vi "Phase III PID.vi"() -> ()   [LabVIEW 2022 SP3]
uses:
  Controls/Notifier data ctl.ctl
  Globals/Phase III Globals.vi
panel:
  out "E_TC_NE":dbl format="%.2g"
  out "E_TC_ET2":dbl format="%.2g"
  out "N_EPV_202_NO":bool
  out "Boolean 92":bool
  out "Boolean 93":bool
  out "Boolean 91":bool
  out "E_PT_CC1":dbl format="%.2g"
  out "E_RTD_NE2":dbl format="%.2g"
  out "E_RTD_NE1":dbl format="%.2g"
  out "E_RTD_ET2":dbl format="%.2g"
  out "E_RTD_ET1":dbl format="%.2g"
  out "E_RTD_TC2":dbl format="%.2g"
  out "E_RTD_TC1":dbl format="%.2g"
  out "Boolean 90":bool
  out "Boolean 89":bool
  out "Boolean 88":bool
  out "F_PT_32":dbl format="%.2g"
  out "C_PT_156":dbl format="%.2g"
  in  "notifier out":refnum<notifier>
  out "F_EPV_136 _NC":bool
  out "F_EPV_41_NC":bool
  out "N_EPV_75_NO":bool
  out "N_EPV_75_NO HS":bool
  out "N_EPV_203_NO":bool
  out "F_EPV_28_NC":bool
  out "F_EPV_1352_NO":bool
  out "N_EPV_62a_NO":bool
  out "C_EPV_7_NC":bool
  out "C_EPV_ 2_NC":bool
  out "F_CMFM_27 (FR)":dbl format="%.2g"
  out "Boolean 87":bool
  out "F_CMFM_43(D)":dbl format="%.2g"
  out "C_CMFM_11 (D)":dbl format="%.2g"
  out "G_CMFM_53 (FR)":dbl format="%.2g"
  out "Boolean 38":bool
  out "C_EPV_ 141_NO HS":bool
  out "N_EPV_69_NO":bool
  out "Boolean 3":bool
  out "N_EPV_68_NO":bool
  out "N_EPV_68_NO HS":bool
  out "Boolean 6":bool
  out "F_EPV_131_NO":bool
  out "Boolean 18":bool
  out "G_EPV_51_NC":bool
  out "C_EPV_ 124_NO":bool
  out "Boolean 13":bool
  out "N_EPV_142_NO":bool
  out "Boolean 41":bool
  out "Boolean 11":bool
  out "Boolean 14":bool
  out "Boolean 29":bool
  out "Boolean 28":bool
  out "Boolean 27":bool
  out "Boolean 26":bool
  out "Boolean 25":bool
  out "Boolean 9":bool
  out "Boolean 7":bool
  out "Boolean 8":bool
  out "Boolean 5":bool
  out "Boolean 6":bool
  out "Boolean 3":bool
  out "Boolean 4":bool
  out "Boolean 24":bool
  out "Boolean 23":bool
  out "Boolean 25":bool
  out "Boolean 26":bool
  out "Boolean 21":bool
  out "N_EPV_61_NO":bool
  out "I_Voltage(V)":dbl format="%.2g"
  out "I_Current(A)":dbl format="%.2g"
  out "Boolean 724":bool
  out "F_CMFM_43(FR)":dbl format="%.2g"
  out "C_PT_45":dbl format="%.2g"
  out "G_CMFM_53(D)":dbl format="%.2g"
  out "C_PT_55":dbl format="%.2g"
  out "C_RTD_20":dbl format="%.2g"
  out "Boolean 18":bool
  out "Boolean 36":bool
  out "Boolean 47":bool
  out "Boolean 4":bool
  out "C_EPV_7_NC HS":bool
  out "Boolean 14":bool
  out "Boolean 19":bool
  out "Boolean 31":bool
  out "Boolean 30":bool
  out "Boolean 24":bool
  out "Boolean 35":bool
  out "Boolean 33":bool
  out "Boolean 34":bool
  out "Boolean 32":bool
  out "Boolean 10":bool
  out "Boolean 11":bool
  out "Boolean 12":bool
  out "Boolean 6":bool
  out "Boolean 45":bool
  out "Boolean 44":bool
  out "Boolean 46":bool
  out "Boolean 42":bool
  out "Boolean 40":bool
  out "Boolean 39":bool
  out "N_EPV_142_NO HS":bool
  out "Boolean 37":bool
  out "Boolean 43":bool
  out "Boolean38":bool
  out "Boolean 7":bool
  out "Boolean 1":bool
  out "Boolean 2":bool
  out "N_EPV_69_NO HS":bool
  out "Boolean 4":bool
  out "Boolean 9":bool
  out "Boolean 5":bool
  out "Boolean 8":bool
  out "Boolean 10":bool
  out "Boolean 11":bool
  out "Boolean 12":bool
  out "Boolean 18":bool
  out "Boolean 13":bool
  out "Boolean 17":bool
  out "Boolean 16":bool
  out "Boolean 19":bool
  out "Boolean 9":bool
  out "Boolean 8":bool
  out "N_EPV_206_NO":bool
  out "Boolean 16":bool
  out "Boolean 15":bool
  out "N_EPV_206_NO HS":bool
  out "Boolean 23":bool
  out "Boolean 22":bool
  out "Boolean 21":bool
  out "Boolean 17":bool
  out "N_EPV_203_NO HS":bool
  out "Boolean 13":bool
  out "Boolean 12":bool
  out "Boolean 27":bool
  out "Boolean 26":bool
  out "Boolean":bool
  out "F_PT_49":dbl format="%.2g"
  out "Boolean 23":bool
  out "Boolean 24":bool
  out "F_EPV_41_NC HS":bool
  out "Boolean 22":bool
  out "Boolean 21":bool
  out "Boolean 20":bool
  out "Boolean 15":bool
  out "Boolean 10":bool
  out "Boolean 1":bool
  out "Boolean 2":bool
  out "I_MPT":dbl format="%.2g"
  out "C_PT_13d":dbl format="%.2g"
  out "C_RTD_13b":dbl format="%.2g"
  out "C_PT_13b":dbl format="%.2g"
  out "Boolean 4":bool
  out "Boolean 18":bool
  out "F_RTD_31a":dbl format="%.2g"
  out "F_PT_31a":dbl format="%.2g"
  out "Boolean 3":bool
  out "Boolean 5":bool
  out "Boolean 2":bool
  out "Boolean 1":bool
  out "E_TC_CC":dbl format="%.2g"
  out "F_RTD_Regen1":dbl format="%.2g"
  out "F_RTD_Regen2":dbl format="%.2g"
  out "E_TC_ET":dbl format="%.2g"
  out "Boolean 9":bool caption="Boolean 6"
  out "Boolean 8":bool
  out "F_PT_29 a":dbl format="%.2g"
  out "F_RTD_29":dbl format="%.2g"
  out "Boolean 7":bool
  out "F_EPV_28_NC HS":bool
  out "F_PT_D":dbl format="%.2g"
  out "Boolean 5":bool
  out "F_PT_SC":dbl format="%.2g"
  out "F_RTD_SC":dbl format="%.2g"
  out "F_PT_S":dbl format="%.2g"
  out "Boolean 4":bool
  out "F_EPV_33_NC":bool
  out "Boolean 3":bool
  out "F_EPV_33_NC HS":bool
  out "F_CMFM_27(D)":dbl format="%.2g"
  out "F_PT_24":dbl format="%.2g"
  out "F_EPV_21_NC":bool
  out "Boolean 2":bool
  out "F_EPV_21_NC HS":bool
  out "Boolean 1":bool
  out "Boolean 14":bool
  out "Boolean 13":bool
  out "F_EPV_132_NO HS":bool
  out "F_EPV_131_NO HS":bool
  out "F_EPV_132_NO":bool
  out "Boolean 20":bool
  out "Boolean 19":bool
  out "Boolean 17":bool
  out "Boolean 16":bool
  out "Boolean 15":bool
  out "Boolean 5":bool
  out "Boolean 4":bool
  out "Boolean 9":bool
  out "Boolean 10":bool
  out "F_PT_129b":dbl format="%.2g"
  out "Boolean 11":bool
  out "Boolean 12":bool
  out "Boolean 8":bool
  out "F_PT_129a":dbl format="%.2g"
  out "F_EPV_136 _NC HS":bool
  out "Boolean 7":bool
  out "Boolean 3":bool
  out "Boolean 6":bool
  out "Boolean 2":bool
  out "F_PT_135":dbl format="%.2g"
  out "Boolean 1":bool
  out "N_EPV_62a_NO HS":bool
  out "Boolean 5":bool
  out "Boolean 71":bool
  out "Boolean 65":bool
  out "Boolean 69":bool
  out "Boolean 68":bool
  out "Boolean 67":bool
  out "Boolean 66":bool
  out "Boolean 70":bool
  out "Boolean 59":bool
  out "Boolean 63":bool
  out "Boolean 62":bool
  out "Boolean 61":bool
  out "Boolean 60":bool
  out "Boolean 64":bool
  out "Boolean 53":bool
  out "Boolean 57":bool
  out "Boolean 56":bool
  out "Boolean 55":bool
  out "Boolean 54":bool
  out "Boolean 58":bool
  out "Boolean 51":bool
  out "Boolean 50":bool
  out "Boolean 49":bool
  out "Boolean 48":bool
  out "Boolean 52":bool
  out "Boolean 76":bool
  out "Boolean 77":bool
  out "Boolean 78":bool
  out "Boolean 80":bool
  out "Boolean 79":bool
  out "Boolean 81":bool
  out "Boolean 9":bool
  out "Boolean 8":bool
  out "Boolean 83":bool
  out "Boolean 82":bool
  out "Boolean 84":bool
  out "C_EPV_ 141_NO":bool
  out "Boolean 85":bool
  out "Boolean 86":bool
  out "N_EPV_62b_NO":bool
  out "Boolean 1":bool
  out "Boolean 2":bool
  out "Boolean 3":bool
  out "Boolean 73":bool
  out "N_EPV_202_NO HS":bool
  out "Boolean 74":bool
  out "Boolean 4":bool
  out "N_EPV_62b_NO HS":bool
  out "Boolean 72":bool
  out "Boolean 75":bool
  out "Boolean 19":bool
  out "Boolean 18":bool
  out "Boolean 20":bool
  out "N_EPV_61_NO HS":bool
  out "Boolean 17":bool
  out "Boolean 16":bool
  out "Boolean 1":bool
  out "Boolean 4":bool
  out "G_EPV_51_NC HS":bool
  out "Boolean 3":bool
  out "Boolean 6":bool
  out "Boolean 2":bool
  out "Boolean 5":bool
  out "G_PT_51":dbl format="%.2g"
  out "Boolean 7":bool
  out "Boolean 11":bool
  out "Boolean 14":bool
  out "Boolean 12":bool
  out "Boolean 10":bool
  out "Boolean 15":bool
  out "Boolean 28":bool
  out "Boolean 22":bool
  out "Boolean 27":bool
  out "Boolean 29":bool
  out "Boolean 30":bool
  out "Boolean 1":bool
  out "Boolean 2":bool
  out "E_TC_inj2":dbl format="%.2g"
  out "I_TC":dbl format="%.2g"
  out "5":dbl format="%.2g"
  out "F_PT_29b":dbl format="%.2g"
  out "F_PT_29c":dbl format="%.2g"
  out "Boolean 840":bool
  out "Boolean 716":bool
  out "Boolean 787":bool
  out "E_PT_CC3":dbl format="%.2g"
  out "E_PT_CC4":dbl format="%.2g"
  out "E_PT_CC5":dbl format="%.2g"
  out "E_PT_CC2":dbl format="%.2g"
  out "F_RTD_31b":dbl format="%.2g"
  out "F_PT_ 31b":dbl format="%.2g"
  out "Boolean 42":bool
  out "Boolean 841":bool
  out "C_PT_13c":dbl format="%.2g"
  out "C_PT_13a":dbl format="%.2g"
  out "C_RTD_13a":dbl format="%.2g"
  out "C_EPV_16_NC":bool
  out "Boolean 15":bool
  out "C_EPV_16_NC HS":bool
  out "Boolean 13":bool
  out "C_PT_D":dbl format="%.2g"
  out "C_EPV_18_NO HS":bool
  out "C_EPV_18_NO":bool
  out "Boolean 16":bool
  out "Boolean 14":bool
  out "C_RTD_17":dbl format="%.2g"
  out "Boolean 17":bool
  out "Boolean 12":bool
  out "Boolean 10":bool
  out "Boolean 11":bool
  out "Boolean 2":bool
  out "Boolean 18":bool
  out "Boolean 838":bool
  out "Boolean 8":bool
  out "N_PT_1351":dbl format="%.2g"
  out "F_EPV_1352_NO HS":bool
  out "Boolean 26":bool
  out "C_PT_SC":dbl format="%.2g"
  out "C_RTD_SC":dbl format="%.2g"
  out "C_PT_S":dbl format="%.2g"
  out "Boolean 7":bool
  out "C_CMFM_11(FR)":dbl format="%.2g"
  out "C_PT_155":dbl format="%.2g"
  out "C_EPV_ 803_NC":bool
  out "Boolean 6":bool
  out "Boolean 5":bool
  out "LOX \n Storage \nTank 2":dbl(slide) scale=0.0..100.0 scale format="%.2f"
  out "C_EPV_ 803_NC HS":bool
  out "C_RTD_5":dbl format="%.2g"
  out "C_EPV_ 8_NC":bool
  out "C_EPV_ 8_NC HS":bool
  out "Boolean 19":bool
  out "Boolean 2":bool
  out "C_EPV_ 2_NC HS":bool
  out "Boolean 1":bool
  out "Boolean 3":bool
  out "LOX \n Storage\nTank 1":dbl(slide) scale=0.0..100.0 scale format="%.2f"
  out "C_EPV_ 123_NO":bool
  out "C_EPV_ 123_NO HS":bool
  out "Boolean 10":bool
  out "C_EPV_ 124_NO HS":bool
  out "Boolean 14":bool
  out "Boolean 9":bool
  out "Boolean 11":bool
  out "Boolean 12":bool
  out "Boolean 8":bool
  out "C_EPV_ 127_NC":bool
  out "Boolean 6":bool
  out "C_EPV_ 127_NC HS":bool
  out "Boolean 5":bool
  out "C_PT_126":dbl format="%.2g"
  out "Boolean 4":bool
  out "Boolean 3":bool
  out "Boolean 1":bool
  out "Boolean 2":bool
  out "ATF Pressure Vessel":dbl(slide) scale=0.0..100.0 scale format="%.2f"
  out "LOX Pressure Vessel":dbl(slide) scale=0.0..100.0 scale format="%.2f"
  # "VERSION NUMBER: 1.1"
  # "PHASE III - PID GUI"
  # "RELEASE DATE: 03/06/24"
  # "ATF\nPressure\n Vessel"
  # "LOX \nPressure\n Vessel"
  # "CH4"
  # "Purge"
  # "N2"
  # "N2"
  # "N24"
  # "N24"
  # "N24"
  # "N24"
  # "N24"
  # "O24"
  # "N24"
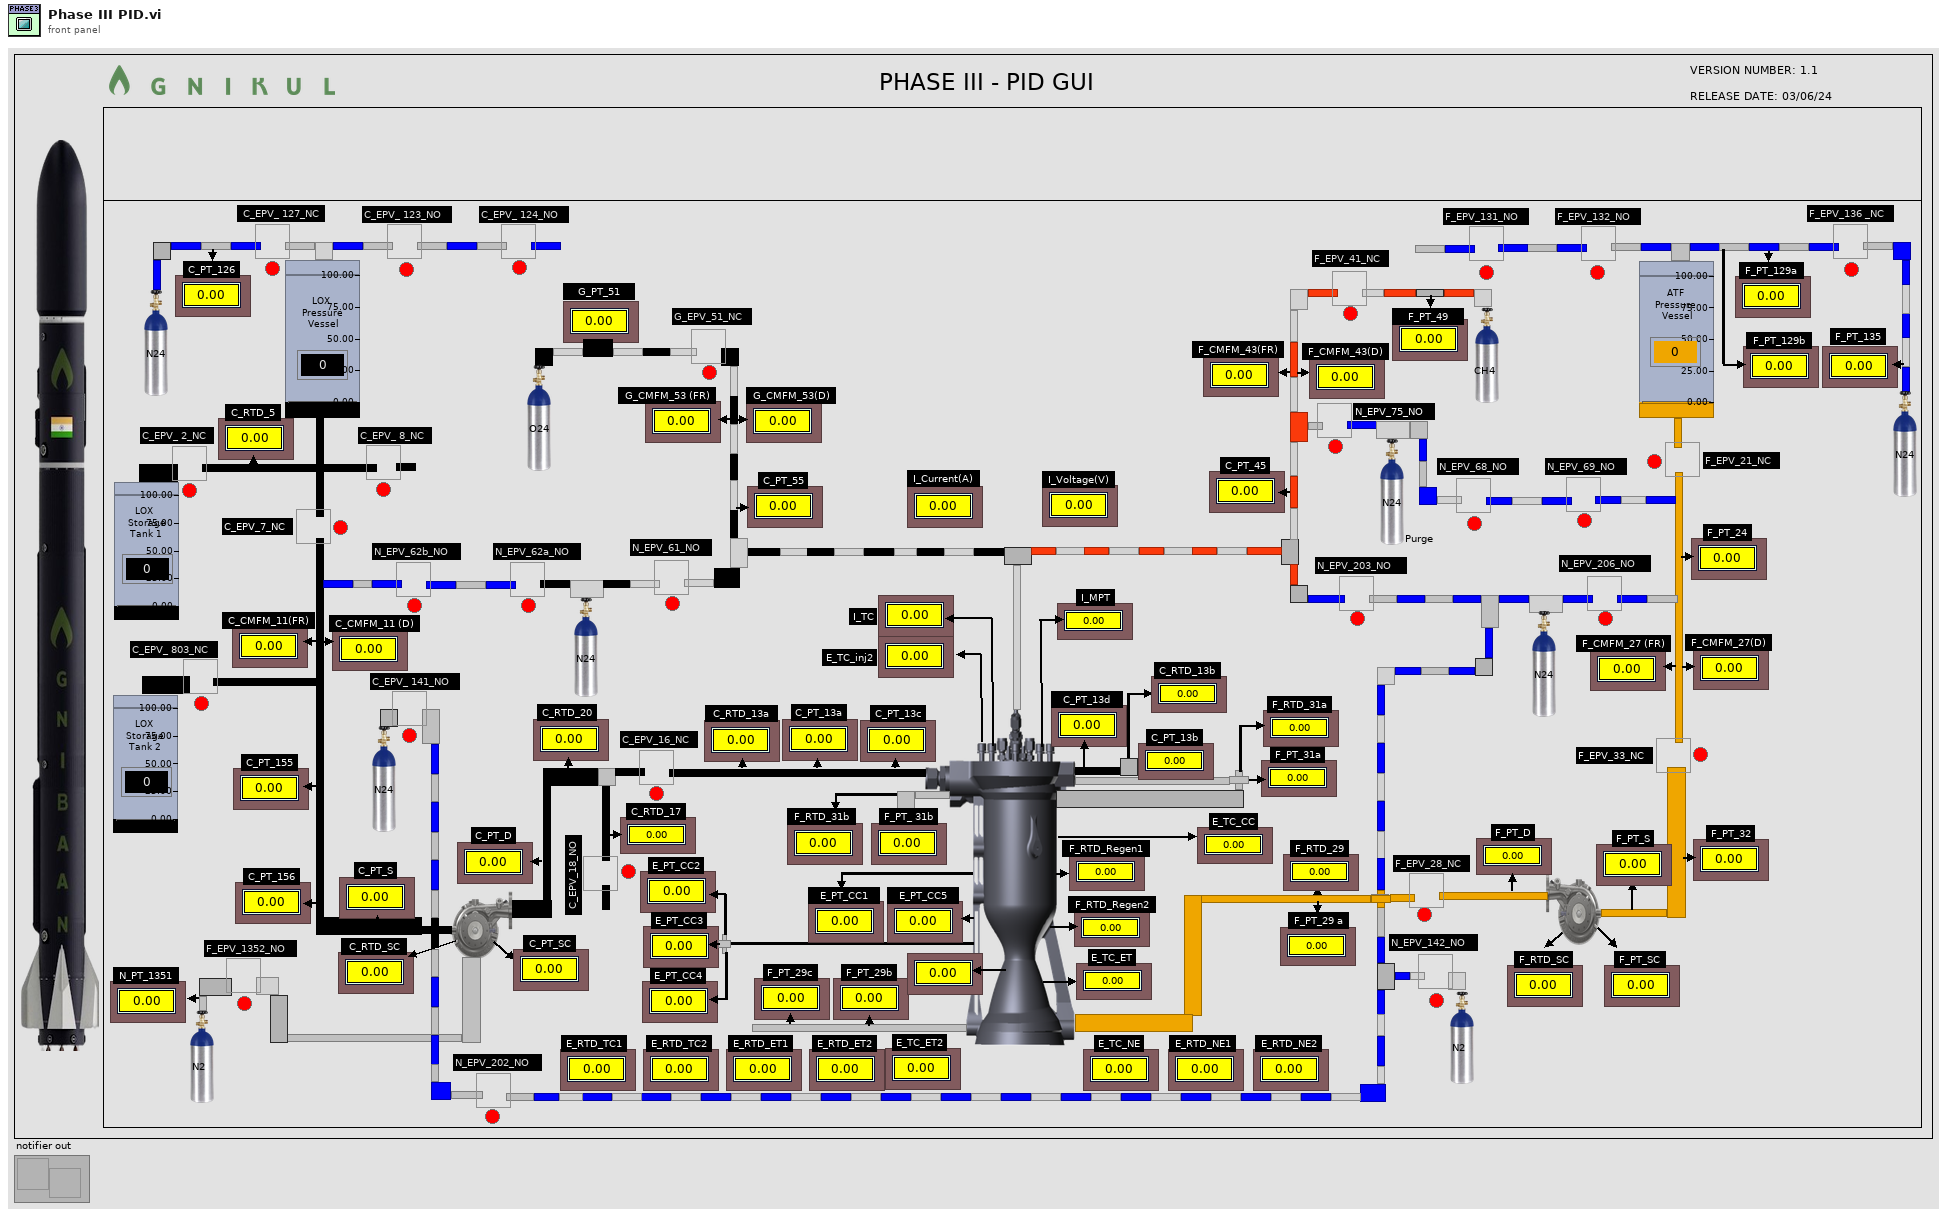
[diagram p1: front panel]
types:
  T1 = cluster{"AI Data":waveform(dbl)[], "DI Data ":digitalwaveform[]}
  T2 = typedef "Notifier data ctl.ctl" = cluster{"Message":string, "Data":variant}
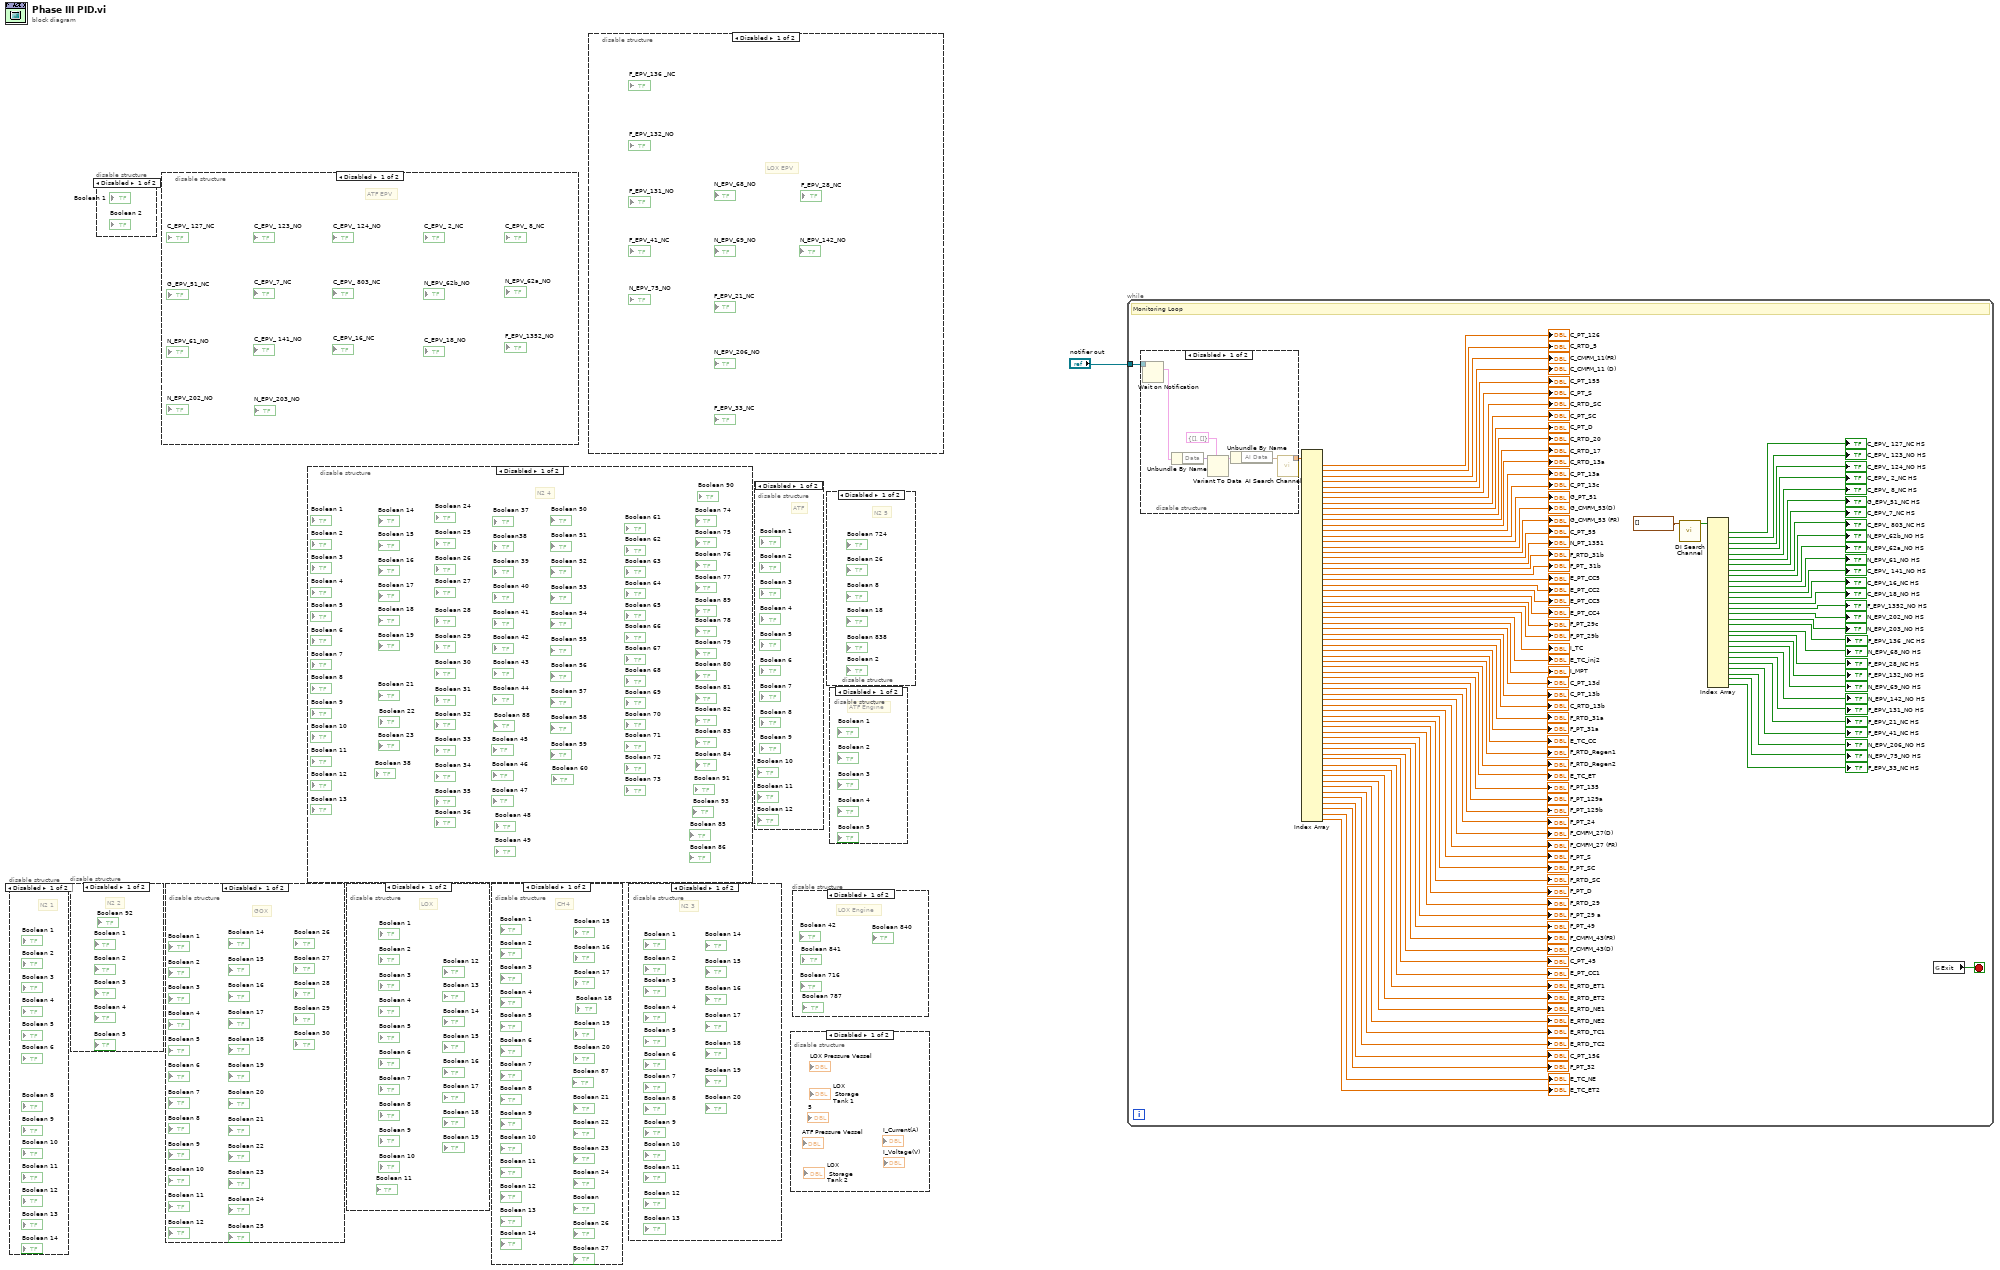
[diagram p0: block diagram]
diagram:
  n1 = disable-structure shown="Disabled" {
    frame Disabled {
      # "N2 1"
    }
    frame Enabled {
    }
  }
  n2 = disable-structure shown="Disabled" {
    frame Disabled {
      # "N2 2"
    }
    frame Enabled {
    }
  }
  n3 = disable-structure shown="Disabled" {
    frame Disabled {
    }
    frame Enabled {
    }
  }
  n4 = disable-structure shown="Disabled" {
    frame Disabled {
      # "ATF EPV"
    }
    frame Enabled {
    }
  }
  n5 = disable-structure shown="Disabled" {
    frame Disabled {
      # "GOX"
    }
    frame Enabled {
    }
  }
  n6 = disable-structure shown="Disabled" {
    frame Disabled {
      # "N2 4"
    }
    frame Enabled {
    }
  }
  n7 = disable-structure shown="Disabled" {
    frame Disabled {
      # "LOX"
    }
    frame Enabled {
    }
  }
  n8 = disable-structure shown="Disabled" {
    frame Disabled {
      # "CH4"
    }
    frame Enabled {
    }
  }
  n9 = disable-structure shown="Disabled" {
    frame Disabled {
      # "LOX EPV"
    }
    frame Enabled {
    }
  }
  n10 = disable-structure shown="Disabled" {
    frame Disabled {
      # "N2 3"
    }
    frame Enabled {
    }
  }
  n11 = disable-structure shown="Disabled" {
    frame Disabled {
      # "ATF"
    }
    frame Enabled {
    }
  }
  n12 = disable-structure shown="Disabled" {
    frame Disabled {
    }
    frame Enabled {
    }
  }
  n13 = disable-structure shown="Disabled" {
    frame Disabled {
      # "LOX Engine"
    }
    frame Enabled {
    }
  }
  n14 = disable-structure shown="Disabled" {
    frame Disabled {
      # "N2 5"
    }
    frame Enabled {
    }
  }
  n15 = disable-structure shown="Disabled" {
    frame Disabled {
      # "ATF Engine"
    }
    frame Enabled {
    }
  }
  n16 = while {
    tunnel: "notifier out" -> [w13]
    stop <- w14 stop-if-true
    # "Monitoring Loop"
    n17 = disable-structure shown="Disabled" {
      disable-tunnel: [w108 _] -> w16
      disable-tunnel: w13 -> [w107 _]
      frame Disabled {
        n18 = Wait on Notification(notifier=w107) -> (notification=w106:T2)  [unwired: 3 in, 3 out]
        n19 = Unbundle By Name(w106) -> ("Data"=w105:variant)
        n20 = Variant To Data(type=T1 {"AI Data"=[], "DI Data "=[]}, Variant=w105) -> (data=w103:T1)  [unwired: 1 in, 1 out]
        n21 = Unbundle By Name(w103) -> ("AI Data"=w102:waveform(dbl)[])
        n22 = call "AI Search Channel.vi"("AI Data"=w102) -> ("FeedBack"=w108:dbl[])  [unwired: 10 in]
      }
      frame Enabled {
      }
    }
    n23 = Index Array(array=w16) -> (element #1=→"C_PT_126":dbl, element #2=→"C_RTD_5":dbl, element #3=→"C_CMFM_11(FR)":dbl, element #4=→"C_CMFM_11 (D)":dbl, element #5=→"C_PT_155":dbl, element #6=→"C_PT_S":dbl, element #7=→"C_RTD_SC":dbl, element #8=→"C_PT_SC":dbl, element #9=→"C_PT_D":dbl, element #10=→"C_RTD_20":dbl, element #11=→"C_RTD_17":dbl, element #12=→"C_RTD_13a":dbl, element #13=→"C_PT_13a":dbl, element #14=→"C_PT_13c":dbl, element #15=→"G_PT_51":dbl, element #16=→"G_CMFM_53(D)":dbl, element #17=→"G_CMFM_53 (FR)":dbl, element #18=→"C_PT_55":dbl, element #19=→"N_PT_1351":dbl, element #20=→"F_RTD_31b":dbl, element #21=→"F_PT_ 31b":dbl, element #22=→"E_PT_CC5":dbl, element #23=→"E_PT_CC2":dbl, element #24=→"E_PT_CC3":dbl, element #25=→"E_PT_CC4":dbl, element #26=→"F_PT_29c":dbl, element #27=→"F_PT_29b":dbl, element #28=→"I_TC":dbl, element #29=→"E_TC_inj2":dbl, element #30=→"I_MPT":dbl, element #31=→"C_PT_13d":dbl, element #32=→"C_PT_13b":dbl, element #33=→"C_RTD_13b":dbl, element #34=→"F_RTD_31a":dbl, element #35=→"F_PT_31a":dbl, element #36=→"E_TC_CC":dbl, element #37=→"F_RTD_Regen1":dbl, element #38=→"F_RTD_Regen2":dbl, element #39=→"E_TC_ET":dbl, element #40=→"F_PT_135":dbl, element #41=→"F_PT_129a":dbl, element #42=→"F_PT_129b":dbl, element #43=→"F_PT_24":dbl, element #44=→"F_CMFM_27(D)":dbl, element #45=→"F_CMFM_27 (FR)":dbl, element #46=→"F_PT_S":dbl, element #47=→"F_PT_SC":dbl, element #48=→"F_RTD_SC":dbl, element #49=→"F_PT_D":dbl, element #50=→"F_RTD_29":dbl, element #51=→"F_PT_29 a":dbl, element #52=→"F_PT_49":dbl, element #53=→"F_CMFM_43(FR)":dbl, element #54=→"F_CMFM_43(D)":dbl, element #55=→"C_PT_45":dbl, element #56=→"E_PT_CC1":dbl, element #57=→"E_RTD_ET1":dbl, element #58=→"E_RTD_ET2":dbl, element #59=→"E_RTD_NE1":dbl, element #60=→"E_RTD_NE2":dbl, element #61=→"E_RTD_TC1":dbl, element #62=→"E_RTD_TC2":dbl, element #63=→"C_PT_156":dbl, element #64=→"F_PT_32":dbl, element #65=→"E_TC_NE":dbl, element #66=→"E_TC_ET2":dbl)  [unwired: 66 in]
    n24 = call "DI Search Channel.vi"("DI Data"=digitalwaveform[] []) -> ("Array 2"=w46:bool[])  [unwired: 10 in]
    n25 = Index Array(array=w46) -> (element #1=→"C_EPV_ 127_NC HS":bool, element #2=→"C_EPV_ 123_NO HS":bool, element #3=→"C_EPV_ 124_NO HS":bool, element #4=→"C_EPV_ 2_NC HS":bool, element #5=→"C_EPV_ 8_NC HS":bool, element #6=→"G_EPV_51_NC HS":bool, element #7=→"C_EPV_7_NC HS":bool, element #8=→"C_EPV_ 803_NC HS":bool, element #9=→"N_EPV_62b_NO HS":bool, element #10=→"N_EPV_62a_NO HS":bool, element #11=→"N_EPV_61_NO HS":bool, element #12=→"C_EPV_ 141_NO HS":bool, element #13=→"C_EPV_16_NC HS":bool, element #14=→"C_EPV_18_NO HS":bool, element #15=→"F_EPV_1352_NO HS":bool, element #16=→"N_EPV_202_NO HS":bool, element #17=→"N_EPV_203_NO HS":bool, element #18=→"F_EPV_136 _NC HS":bool, element #19=→"N_EPV_68_NO HS":bool, element #20=→"F_EPV_28_NC HS":bool, element #21=→"F_EPV_132_NO HS":bool, element #22=→"N_EPV_69_NO HS":bool, element #23=→"N_EPV_142_NO HS":bool, element #24=→"F_EPV_131_NO HS":bool, element #25=→"F_EPV_21_NC HS":bool, element #26=→"F_EPV_41_NC HS":bool, element #27=→"N_EPV_206_NO HS":bool, element #28=→"N_EPV_75_NO HS":bool, element #29=→"F_EPV_33_NC HS":bool)  [unwired: 29 in]
    n26 = global read "Phase III Globals.vi" "Exit"() -> (w14:bool)
  }
